vi "Create Room Service Request.vi"(0 "Hotel Management Tool Model in":refnum<class "Hotel Management Tool Model.lvclass">, 5 "Rooms No":string, 7 "Room Service":refnum<class "Room Service Base.lvclass">, 11 "error in (no error)":errorcluster) -> (4 "Hotel Management Tool Model out":refnum<class "Hotel Management Tool Model.lvclass">, 15 "error out":errorcluster)   [LabVIEW 2023, in "Hotel Management Tool Model.lvlib" / "Hotel Management Tool Model.lvclass"]
uses:
  Hotel Management Tool Model.lvclass
  Hotel Management Tool Model.lvclass/Hotel Management Tool Model.ctl
  Central Data Manager/Central Data Manager Messages/Create Room Service Request Msg/Create Room Service Request Msg.lvclass
  Room Service Types/Room Service Base/Room Service Base.lvclass
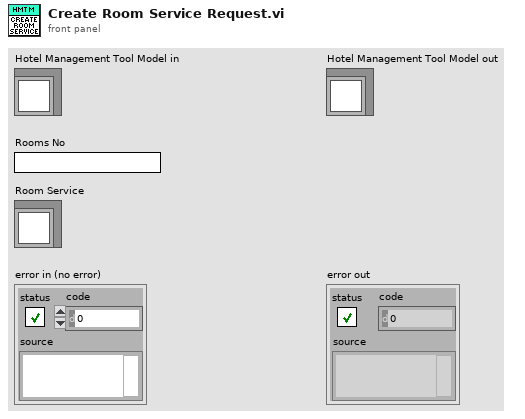
[diagram p1: front panel]
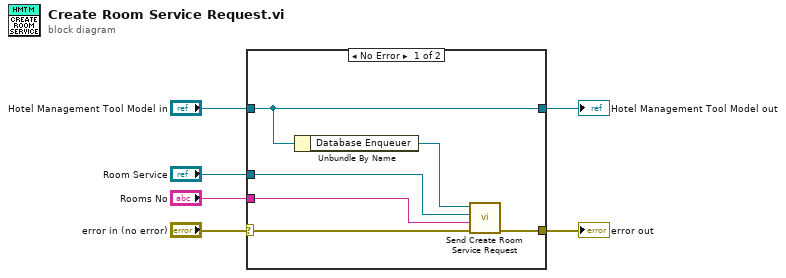
[diagram p0: block diagram]
diagram:
  n1 = case shown="No Error" "error in (no error)" {
    selector: "error in (no error)" -> [w11 w14]
    tunnel: [w10 w14] -> w3
    tunnel: [w12 w13] -> w5
    tunnel: "Hotel Management Tool Model in" -> [w12 w13]
    tunnel: "Room Service" -> [w7 _]
    tunnel: "Rooms No" -> [w8 _]
    frame No Error {
      n2 = Unbundle By Name(w12) -> ("Database Enqueuer"=w9:refnum<class "Message Enqueuer.lvclass">)
      n3 = call "Send Create Room Service Request.vi"("error in (no error)"=w11, "Rooms No"=w8, "Room Service"=w7, "Message Enqueuer"=w9) -> ("error out"=w10:errorcluster)  [unwired: 6 in, 1 out]
    }
    frame Error {
    }
  }
  "error out" <- w3
  "Hotel Management Tool Model out" <- w5
